vi "Convert Steering Frame Velocity to Global.vi"(10 "steering frame angle (rad)":dbl, 11 "steering frame velocity":dbl[](array[numeric])) -> (3 "global velocity":dbl[](array[numeric]))   [LabVIEW 2017, in "NI_Robotics_Steering Frame.lvclass"]
uses:
  <vilib>/robotics/Steering/Steering Frame/NI_Robotics_Steering Frame.lvclass
  <vilib>/Analysis/coordinate.llb/2D Cartesian Coordinate Rotation (Scalar).vi
  <vilib>/Analysis/NI_AALPro.lvlib
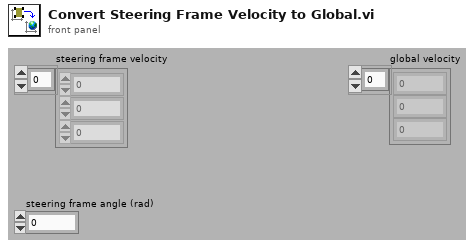
[diagram p1: front panel]
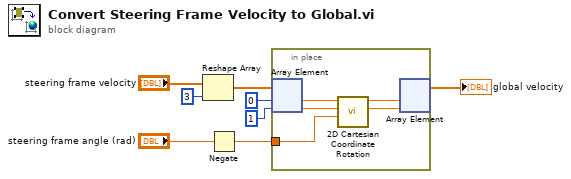
[diagram p0: block diagram]
diagram:
  n1 = Reshape Array("steering frame velocity", 3 ("dimension size")) -> (w6:dbl[])
  n2 = Negate(x="steering frame angle (rad)") -> (-x=w1:dbl)
  n3 = in-place {
    in-place-border: w1 -> [w9]
    n4 = in-place-array #1(w6, 0, 1) -> (w13:dbl, w12:dbl)
    n5 = call-poly <vilib>:"2D Cartesian Coordinate Rotation.vi"("theta"=w9, "y"=w12, "x"=w13) -> ("y out"=w10:dbl, "x out"=w11:dbl)  [unwired: 6 in, 1 out]
    n6 = in-place-array #1(w11, w10) -> (→"global velocity":dbl[])  [unwired: 2 out]
  }
